vi "Get lines from string.vi"(2 "Cut spaces?":bool, 3 "Array size":i32, 4 "Input string":string) -> (15 "Strings":string[](array[string]), 16 "Array size out":i32)   [LabVIEW 2020]
doc: "This VI returns single lines from input string. If number of lines (Array size) is known, algorithm is faster, otherwise Array size = 0 should be used. Sub-VI for VST?.vi and Define macro contents (with or without) delay.vi."
panel:
  # "This vi returns single lines from input string. If number of lines (Array size) is \nknown, algorithm is faster, otherwise Array size = 0 should be used."
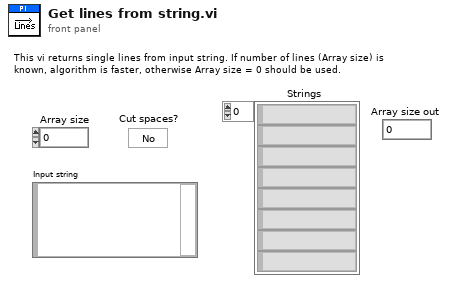
[diagram p1: front panel]
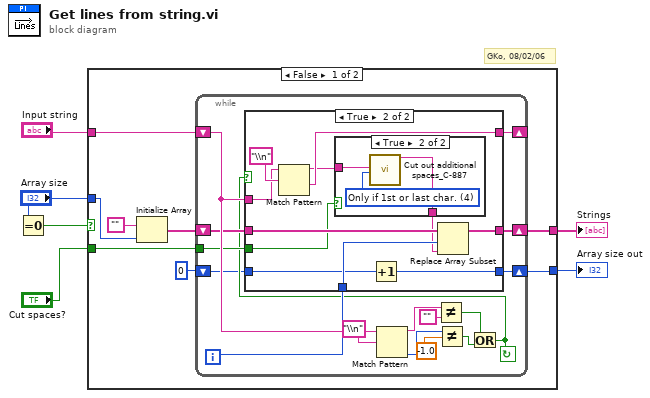
[diagram p0: block diagram]
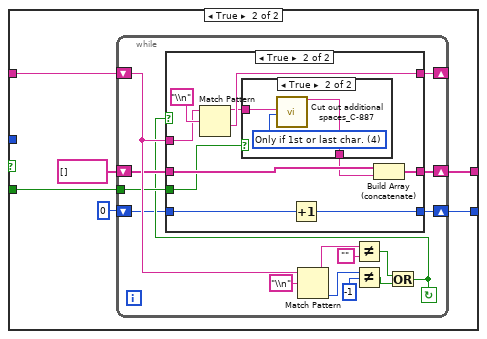
[diagram p4: hidden frame]
diagram:
  # "GKo, 08/02/06"
  n1 = Equal To 0?(x="Array size") -> (x = 0?=w3:bool)
  n2 = case shown="False" w3 {
    tunnel: "Input string" -> [w14 w54]
    tunnel: "Array size" -> [w11 _]
    tunnel: [w10 w53] -> w4
    tunnel: "Cut spaces?" -> [w9 w51]
    tunnel: [w7 w50] -> w1
    frame False {
      n3 = Initialize Array("", w11) -> (w13:string[])
      n4 = while {
        shift-left: w13 -> [w23]
        shift-right: [w24] -> w10
        shift-left: w14 -> [w27]
        shift-right: [w26] -> _
        tunnel: w9 -> [w22]
        shift-right: [w16] -> w7
        shift-left: 0 -> [w15]
        i -> [w25]
        stop <- w20 continue-if-true
        n5 = Match Pattern(string=w27, regular expression="\\n") -> (before substring=w18:string, offset past match=w28:i32)  [unwired: 3 out]
        n6 = Not Equal?(x=w18, y="") -> (x != y?=w19:bool)
        n7 = Not Equal?(x=w28, y=-1.0) -> (x != y?=w21:bool)
        n8 = Or(x=w19, y=w21) -> (x .or. y?=w20:bool)
        n9 = case shown="True" w20 {
          tunnel: w27 -> [w33 w43]
          tunnel: [w33 w42] -> w26
          tunnel: w25 -> [_ w39]
          tunnel: [w32 w41] -> w24
          tunnel: w23 -> [w32 w40]
          tunnel: w22 -> [_ w36]
          tunnel: [w31 w34] -> w16
          tunnel: w15 -> [w31 w35]
          frame False {
          }
          frame True {
            n10 = Match Pattern(string=w43, regular expression="\\n") -> (before substring=w38:string, after substring=w42:string)  [unwired: 3 out]
            n11 = case shown="True" w36 {
              tunnel: w38 -> [w45 w48]
              tunnel: [w45 w47] -> w37
              frame False {
              }
              frame True {
                w46 = u16 4 items=["All Spaces", "Only if 1st char.", "Only if last char.", "Only if near \"=\"", "Only if 1st or last char.", "Only multiple"] ("Mode")
                n12 = call "Cut out additional spaces_C-887.vi"("String"=w48, "Mode"=w46) -> ("String out"=w47:string)  [unwired: 17 out]
              }
            }
            n13 = Increment(x=w35) -> (x+1=w34:i32)
            n14 = Replace Array Subset(array=w40, new element=w37, index=w39) -> (w41:string[])
          }
        }
      }
    }
    frame True {
      n15 = while {
        shift-left: string[] [] -> [w63]
        shift-right: [w64] -> w53
        shift-left: w54 -> [w66]
        shift-right: [w65] -> _
        tunnel: w51 -> [w62]
        shift-right: [w56] -> w50
        shift-left: 0 -> [w55]
        stop <- w59 continue-if-true
        n16 = Match Pattern(string=w66, regular expression="\\n") -> (before substring=w57:string, offset past match=w67:i32)  [unwired: 3 out]
        n17 = Not Equal?(x=w57, y="") -> (x != y?=w61:bool)
        n18 = Not Equal?(x=w67, y=-1) -> (x != y?=w58:bool)
        n19 = Or(x=w61, y=w58) -> (x .or. y?=w59:bool)
        n20 = case shown="True" w59 {
          tunnel: w66 -> [w72 w81]
          tunnel: [w72 w80] -> w65
          tunnel: [w71 w79] -> w64
          tunnel: w63 -> [w71 w78]
          tunnel: w62 -> [_ w75]
          tunnel: [w70 w73] -> w56
          tunnel: w55 -> [w70 w74]
          frame False {
          }
          frame True {
            n21 = Match Pattern(string=w81, regular expression="\\n") -> (before substring=w77:string, after substring=w80:string)  [unwired: 3 out]
            n22 = case shown="True" w75 {
              tunnel: w77 -> [w83 w86]
              tunnel: [w83 w85] -> w76
              frame False {
              }
              frame True {
                w84 = u16 4 items=["All Spaces", "Only if 1st char.", "Only if last char.", "Only if near \"=\"", "Only if 1st or last char.", "Only multiple"] ("Mode")
                n23 = call "Cut out additional spaces_C-887.vi"("String"=w86, "Mode"=w84) -> ("String out"=w85:string)  [unwired: 17 out]
              }
            }
            n24 = Increment(x=w74) -> (x+1=w73:i32)
            n25 = Build Array (concatenate)(w78, w76) -> (w79:string[])
          }
        }
      }
    }
  }
  "Strings" <- w4
  "Array size out" <- w1
